vi "Write Instrument driver.vi"(8 "error in (no error)":errorcluster, 10 "Instrument Driver.lvclass":refnum<class "Instrument Driver.lvclass">, 11 "Instrument Recorder in":refnum<class "Instrument Recorder.lvclass">) -> (0 "error out":errorcluster, 3 "Instrument Recorder out":refnum<class "Instrument Recorder.lvclass">)   [LabVIEW 2015, in "Instrument Recorder.lvclass"]
uses:
  Instrument Recorder.lvclass
  NHMFL_Core/Libraries/Instruments/Instrument Driver/Instrument Driver.lvclass
  Instrument Recorder.lvclass/Instrument Recorder.ctl
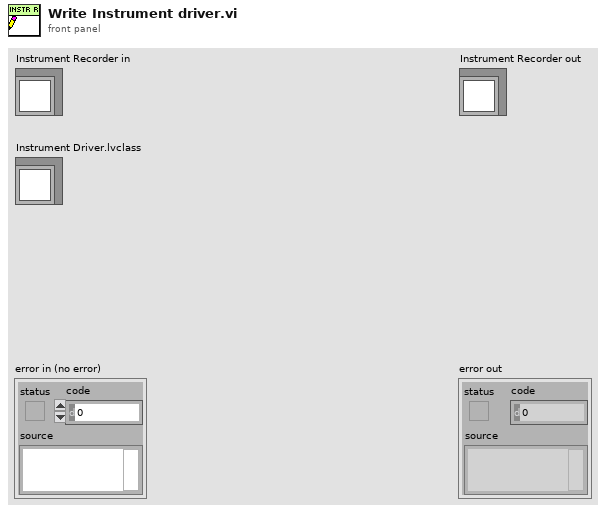
[diagram p1: front panel]
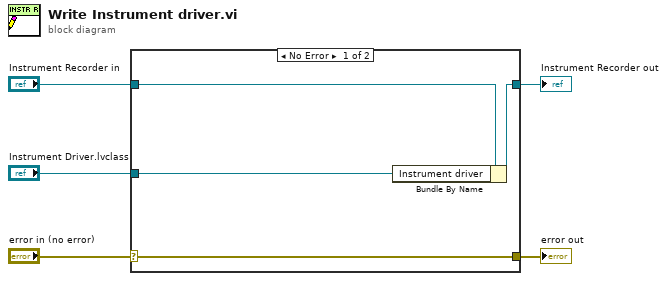
[diagram p0: block diagram]
diagram:
  n1 = case shown="No Error" "error in (no error)" {
    selector: "error in (no error)" -> [w9 w10]
    tunnel: [w9 w10] -> w4
    tunnel: [w7 w11] -> w2
    tunnel: "Instrument Recorder in" -> [w8 w11]
    tunnel: "Instrument Driver.lvclass" -> [w6 _]
    frame No Error {
      n2 = Bundle By Name(cluster=w8, "Instrument driver"=w6) -> (w7:refnum<class "Instrument Recorder.lvclass">)
    }
    frame Error {
    }
  }
  "error out" <- w4
  "Instrument Recorder out" <- w2
